vi "sub_qam_demod.vi"(8 "symbol map":cdb[](array[numeric]), 11 "symbol":cdb[](array[numeric])) -> (3 "bitstream":i16[](array[numeric]))   [LabVIEW 2014]
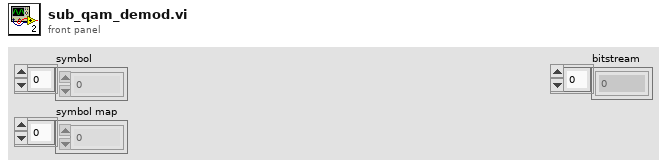
[diagram p1: front panel]
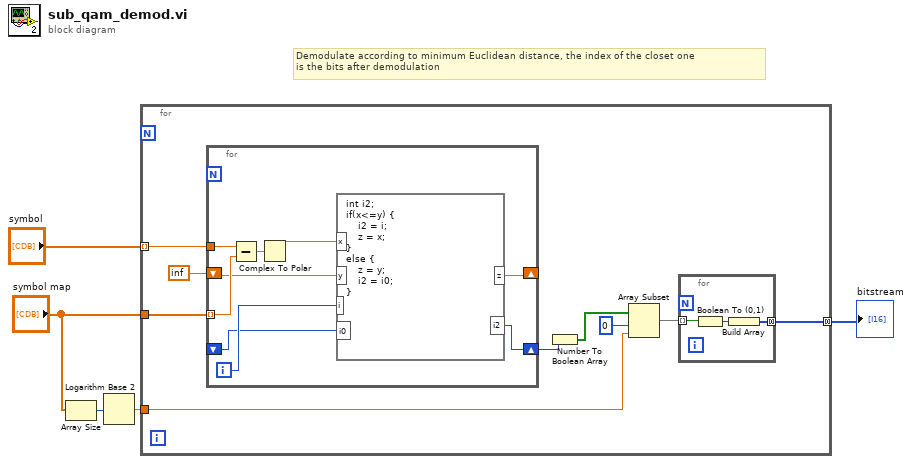
[diagram p0: block diagram]
diagram:
  # "Demodulate according to minimum Euclidean distance, the index of the closet one \nis the bits after demodulation"
  n1 = Array Size(array="symbol map") -> (size(s)=w2:i32)
  n2 = Logarithm Base 2(1:w2) -> (0:w1:dbl)
  n3 = for {
    tunnel: "symbol" -> [w14] mode=indexing
    tunnel: "symbol map" -> [w13]
    tunnel: w1 -> [w8]
    tunnel: [w7] -> w3 mode=concatenating
    n4 = for {
      tunnel: w14 -> [w26]
      tunnel: w13 -> [w25] mode=indexing
      shift-right: [w20] -> w9
      shift-left: _ -> [w21]
      shift-right: [w19] -> _
      shift-left: inf -> [w18]
      i -> [w22]
      n5 = Subtract(x=w26, y=w25) -> (x-y=w24:cdb)
      n6 = Complex To Polar(r * e^(i*theta)=w24) -> (r=w23:dbl)  [unwired: 1 out]
      n7 = formula code="int i2;\nif(x<=y) {\n    i2 = i;\n    z = x;\n}\nelse {\n    z = y;\n    i2 = i0;\n}"("x"=w23, "y"=w18, "i"=w22, "i0"=w21) -> ("z"=w19:dbl, "i2"=w20:i32)
    }
    n8 = Number To Boolean Array(number=w9) -> (Boolean array=w12:bool[])
    n9 = Array Subset(array=w12, index=0, length=w8) -> (w10:bool[])
    n10 = for {
      tunnel: w10 -> [w17] mode=indexing
      tunnel: [w15] -> w7 mode=concatenating
      n11 = Boolean To (0,1)(Boolean=w17) -> (0, 1=w16:i16)
      n12 = Build Array(w16) -> (w15:i16[])
    }
  }
  "bitstream" <- w3
